vi "Execute Command.vi"(8 "error in (no error)":errorcluster, 10 "Command":refnum<class "Command.lvclass">, 11 "Command Handler in":refnum<class "Command Handler.lvclass">) -> (0 "error out":errorcluster, 2 "Stop":bool, 3 "Command Handler out":refnum<class "Command Handler.lvclass">)   [LabVIEW 2015, in "Command Handler.lvlib" / "Command Handler.lvclass"]
uses:
  Command Handler.lvclass
  Command Handler Messages/Command Handler Global API/Command Handler Global.vi
  Command Handler.lvlib
  Command Parent/Command.lvclass
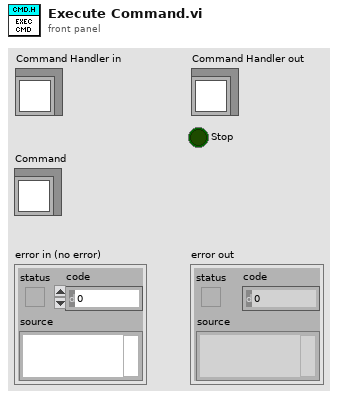
[diagram p1: front panel]
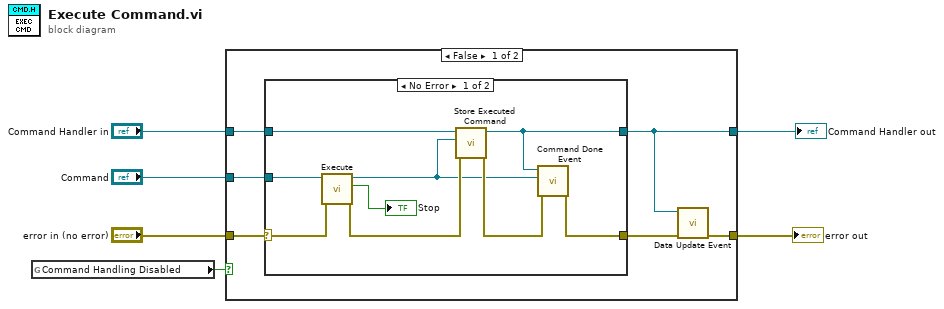
[diagram p0: block diagram]
diagram:
  n1 = global read "Command Handler Global.vi" "Command Handling Disabled"() -> (w1:bool)
  n2 = case shown="False" w1 {
    tunnel: "error in (no error)" -> [w12 w24]
    tunnel: "Command Handler in" -> [w11 w25]
    tunnel: "Command" -> [w10 _]
    tunnel: [w9 w24] -> w3
    tunnel: [w8 w25] -> w2
    frame False {
      n3 = case shown="No Error" w12 {
        selector: w12 -> [w19 w23]
        tunnel: [w16 w23] -> w7
        tunnel: [w13 w22] -> w8
        tunnel: w11 -> [w21 w22]
        tunnel: w10 -> [w20 _]
        frame No Error {
          n4 = call-dynamic "Execute.vi"("error in (no error)"=w19, "Command in"=w20) -> ("error out"=w18:errorcluster, "Stop"=→"Stop":bool, "Command out"=w14:refnum<class "Command.lvclass">)  [unwired: 7 in]
          n5 = call-dynamic "Store Executed Command.vi"("error in (no error)"=w18, "Completed Command"=w14, "Command Handler in"=w21) -> ("error out"=w15:errorcluster, "Command Handler out"=w13:refnum<class "Command Handler.lvclass">)  [unwired: 7 in]
          n6 = call "Command Done Event.vi"("error in (no error)"=w15, "Command In"=w14, "Command Handler in"=w13) -> ("error out"=w16:errorcluster)  [unwired: 8 in]
        }
        frame Error {
        }
      }
      n7 = call "Data Update Event.vi"("error in (no error)"=w7, "Command Handler in"=w8) -> ("error out"=w9:errorcluster)  [unwired: 9 in]
    }
    frame True {
    }
  }
  "error out" <- w3
  "Command Handler out" <- w2
